vi "Transient Capture - Configure Settings.vi"(6 "DEMUX on UUT":bool, 7 "Soft Trigger":bool=TRUE, 8 "error in":errorcluster, 9 "Samples to Read (Post Trigger)":i32=100000, 10 "Samples to Read (Pre Trigger)":i32=100000, 11 "Carrier Configuration":T1={"Name"="Default Settings", "IP"="192.168.0.84", "Control Port"=4220, "Timeout (ms)"=2000, "Continuous Capture Port (Multiplexed)"=4210, "Start HIL Shot Port"=53999, "AWG Upload Port (Multiplexed)"=54201, "Download Captured Data Port (Multiplexed)"=53000, "Module Slots"=2, "Module Configurations"=[{"Name"="ACQ 425 ELF", "Position"="192.168.0.84", "Module Type"=enum."Analog In Module", "Control Port"=4221, "Timeout (ms)"=2000, "Channels"=16}, {"Name"="AO 424 ELF", "Position"="192.168.0.84", "Module Type"=enum."Analog Out Module", "Control Port"=4222, "Timeout (ms)"=2000, "Channels"=16}]}) -> (0 "error out":errorcluster, 1 "Carrier Connection Out":T4={"Description"="", "Address"="", "Port"=0, "timeout (ms)"=5000, "Termination Character"="\n", "TCP Connection Reference"=refnum, "Open Connection"=FALSE}, 2 "AI Connection Out":T4={"Description"="", "Address"="", "Port"=0, "timeout (ms)"=5000, "Termination Character"="\n", "TCP Connection Reference"=refnum, "Open Connection"=FALSE})   [LabVIEW 2017, in "Communications Library.lvlib"]
doc: "Configures the DTACQ device for transient capture mode.\n\nSets the transient capture mode, trigger mode and event settings."
uses:
  Communications Library.lvlib
  Typedefs/DTACQ Connection Data--Cluster.ctl
  Typedefs/DTACQ Module Carrier Configuration--Cluster.ctl
  Typedefs/DTACQ Module Configuration--Cluster.ctl
  Typedefs/DTACQ Device Type--Enum.ctl
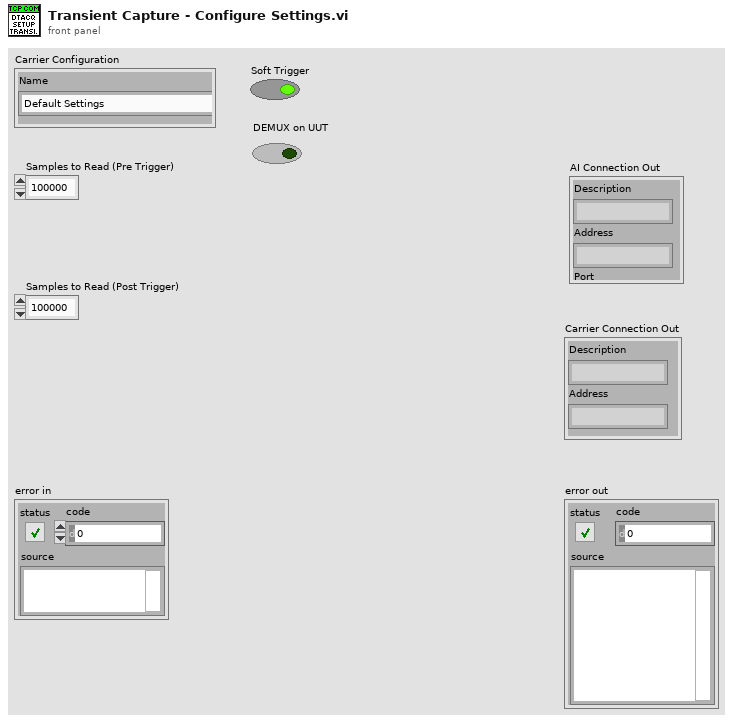
[diagram p1: front panel]
types:
  T1 = typedef "Communications Library.lvlib/DTACQ Module Carrier Configuration--Cluster.ctl" = cluster{"Name":string, "IP":string, "Control Port":i32, "Timeout (ms)":i32, "Continuous Capture Port (Multiplexed)":i32, "Start HIL Shot Port":i32, "AWG Upload Port (Multiplexed)":i32, "Download Captured Data Port (Multiplexed)":i32, "Module Slots":i32, "Module Configurations":T2[]}
  T2 = typedef "Communications Library.lvlib/DTACQ Module Configuration--Cluster.ctl" = cluster{"Name":string, "Position":string, "Module Type":T3, "Control Port":i32, "Timeout (ms)":i32, "Channels":i32}
  T3 = typedef "Communications Library.lvlib/DTACQ Device Type--Enum.ctl" = enum16{"Carrier", "Analog In Module", "Analog Out Module", "Generic Module"}
  T4 = typedef "Communications Library.lvlib/DTACQ Connection Data--Cluster.ctl" = cluster{"Description":string, "Address":string, "Port":u16, "timeout (ms)":i32, "Termination Character":string, "TCP Connection Reference":refnum<k5>, "Open Connection":bool}
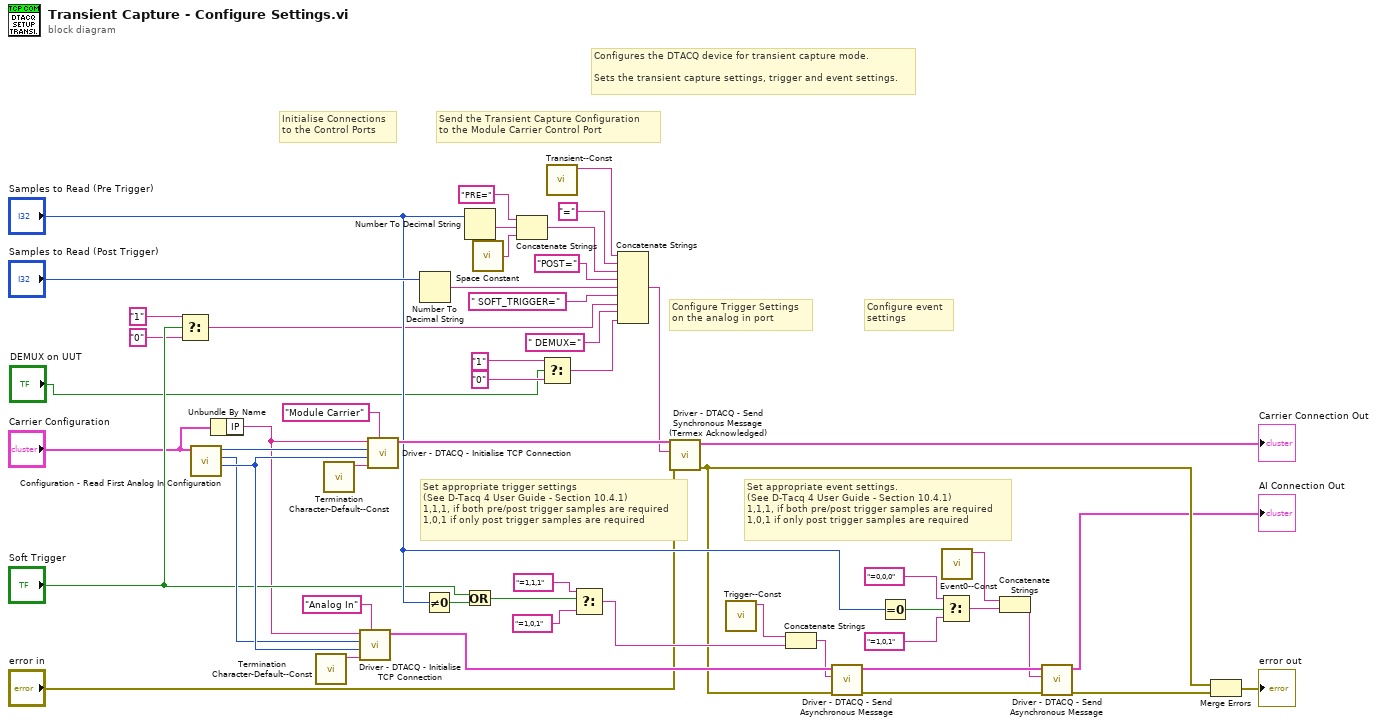
[diagram p0: block diagram]
diagram:
  # "Configure event\nsettings"
  # "Set appropriate event settings.\n(See D-Tacq 4 User Guide - Section 10.4.1)\n1,1,1, if both pre/post trigger samples are required\n1,0,1 if only post trigger samples are required"
  # "Set appropriate trigger settings\n(See D-Tacq 4 User Guide - Section 10.4.1)\n1,1,1, if both pre/post trigger samples are required\n1,0,1 if only post trigger samples are required"
  # "Configures the DTACQ device for transient capture mode.\n\nSets the transient capture settings, trigger and event settings."
  # "Configure Trigger Settings\non the analog in port"
  # "Send the Transient Capture Configuration\nto the Module Carrier Control Port"
  # "Initialise Connections\nto the Control Ports"
  n1 = Select(t="1", s="Soft Trigger", f="0") -> (s? t:f=w8:string)
  n2 = call "Configuration - Read First Analog In Configuration.vi"("Carrier Configuration"="Carrier Configuration") -> ("Timeout (ms)"=w22:i32, "Analog In Control Port"=w21:i32, "Carrier Control Port"=w40:i32)  [unwired: 6 in, 2 out]
  n3 = Unbundle By Name("Carrier Configuration") -> ("IP"=w5:string)
  n4 = call "Termination Character-Default--Const.vi"() -> ("Termination Character"=w48:string)  [unwired: 11 in]
  n5 = call "Termination Character-Default--Const.vi"() -> ("Termination Character"=w50:string)  [unwired: 11 in]
  n6 = call "Driver - DTACQ - Initialise TCP Connection.vi"("Description"="Analog In", "Termination Character"=w48, "timeout (ms)"=w22, "Port"=w21, "Address"=w5) -> ("DTACQ Connection Data Out"=w53:T4)  [unwired: 6 in]
  n7 = call "Driver - DTACQ - Initialise TCP Connection.vi"("Description"="Module Carrier", "Termination Character"=w50, "timeout (ms)"=w22, "Port"=w40, "Address"=w5) -> ("DTACQ Connection Data Out"=w42:T4)  [unwired: 6 in]
  n8 = Number To Decimal String(number="Samples to Read (Post Trigger)") -> (decimal integer string=w47:string)  [unwired: 1 in]
  n9 = Not Equal To 0?(x="Samples to Read (Pre Trigger)") -> (x != 0?=w19:bool)
  n10 = Number To Decimal String(number="Samples to Read (Pre Trigger)") -> (decimal integer string=w35:string)  [unwired: 1 in]
  n11 = Or(x="Soft Trigger", y=w19) -> (x .or. y?=w18:bool)
  n12 = call <vilib>:"Space Constant.vi"() -> ("String"=w34:string)
  n13 = Concatenate Strings("PRE=" ("string"), w35, w34) -> (w37:string)
  n14 = Select(t="1", s="DEMUX on UUT", f="0") -> (s? t:f=w4:string)
  n15 = call "Transient--Const.vi"() -> ("Transient Command"=w39:string)  [unwired: 11 in]
  n16 = Select(t="=1,1,1" ("string"), s=w18, f="=1,0,1" ("string")) -> (s? t:f=w33:string)
  n17 = Concatenate Strings(w39, "=" ("string"), w37, "POST=" ("string"), w47, " SOFT_TRIGGER=" ("string"), w8, " DEMUX=", w4) -> (w41:string)
  n18 = call "Driver - DTACQ - Send Synchronous Message (Termex Acknowledged).vi"("error in"="error in", "Message to Send"=w41, "DTACQ Connection Data In"=w42) -> ("error out"=w15:errorcluster, "DTACQ Connection Data Out"=→"Carrier Connection Out":T4)  [unwired: 5 in, 2 out]
  n19 = call "Trigger--Const.vi"() -> ("Trigger Command"=w44:string)  [unwired: 11 in]
  n20 = Concatenate Strings(w44, w33) -> (w43:string)
  n21 = call "Driver - DTACQ - Send Asynchronous Message.vi"("error in"=w15, "Message to Send"=w43, "DTACQ Connection Data In"=w53) -> ("error out"=w27:errorcluster, "DTACQ Connection Data Out"=w28:T4)  [unwired: 7 in]
  n22 = Equal To 0?(x="Samples to Read (Pre Trigger)") -> (x = 0?=w25:bool)
  n23 = Select(t="=0,0,0" ("string"), s=w25, f="=1,0,1" ("string")) -> (s? t:f=w29:string)
  n24 = call "Event0--Const.vi"() -> ("Event Command"=w32:string)  [unwired: 11 in]
  n25 = Concatenate Strings(w32, w29) -> (w24:string)
  n26 = call "Driver - DTACQ - Send Asynchronous Message.vi"("error in"=w27, "Message to Send"=w24, "DTACQ Connection Data In"=w28) -> ("error out"=w13:errorcluster, "DTACQ Connection Data Out"=→"AI Connection Out":T4)  [unwired: 7 in]
  n27 = Merge Errors(w15, w13) -> (→"error out":errorcluster)
